vi "test Data Width and Data Loss Error.vi"(8 "error in (no error)":errorcluster, 11 "TestCase in":refnum<class "BCD.lvclass">) -> (0 "error out":errorcluster, 3 "TestCase out":refnum<class "BCD.lvclass">)   [LabVIEW 2020, in "BCD.lvclass"]
uses:
  BCD.lvclass
  e4b8c782-df88-4a73-9bfb-bbb124582f89.vi
  e994315a-18d4-4c7c-aace-f9d3bec48076.vi
  3423ebfb-ba8f-439c-a507-83e880fcea0a.vi
  5f41c702-736d-46cb-8ad7-d7a8da9834e5.vi
  e4b8c782-df88-4a73-9bfb-bbb124582f89.vi/a54b505c-1216-4ef4-8378-3ceda9d188df.vi
  e4b8c782-df88-4a73-9bfb-bbb124582f89.vi/136dcdcb-2dd3-4a4d-a796-a8f7a3f8e1ac.vi
  e994315a-18d4-4c7c-aace-f9d3bec48076.vi/0a001d06-2809-4638-8d0b-e017d2157007.vi
  BCD Decode Integer.vi
  3423ebfb-ba8f-439c-a507-83e880fcea0a.vi/a54b505c-1216-4ef4-8378-3ceda9d188df.vi
  3423ebfb-ba8f-439c-a507-83e880fcea0a.vi/136dcdcb-2dd3-4a4d-a796-a8f7a3f8e1ac.vi
  5f41c702-736d-46cb-8ad7-d7a8da9834e5.vi/a54b505c-1216-4ef4-8378-3ceda9d188df.vi
  5f41c702-736d-46cb-8ad7-d7a8da9834e5.vi/136dcdcb-2dd3-4a4d-a796-a8f7a3f8e1ac.vi
  e4b8c782-df88-4a73-9bfb-bbb124582f89.vi/a54b505c-1216-4ef4-8378-3ceda9d188df.vi/a7fcce85-1f75-4572-aeaa-ddfd463a7c5f.vi
  BCD Decode Integer.vi/9a65bfc0-0d77-4ef3-ab58-63df1e1caa90.vi
  3423ebfb-ba8f-439c-a507-83e880fcea0a.vi/a54b505c-1216-4ef4-8378-3ceda9d188df.vi/a7fcce85-1f75-4572-aeaa-ddfd463a7c5f.vi
  5f41c702-736d-46cb-8ad7-d7a8da9834e5.vi/a54b505c-1216-4ef4-8378-3ceda9d188df.vi/a7fcce85-1f75-4572-aeaa-ddfd463a7c5f.vi
  <vilib>/addons/_JKI Toolkits/VI Tester/TestCase.llb/TestCase.lvclass
  C:/Program Files (x86)/National Instruments/LabVIEW 2020/vi.lib/addons/_JKI Toolkits/VI Tester/TestCase.llb/TestCase.lvclass
panel:
  out "BCD encoded value":bool[](array[boolean])
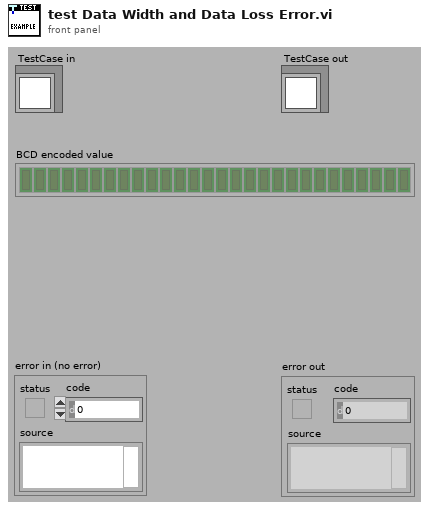
[diagram p1: front panel]
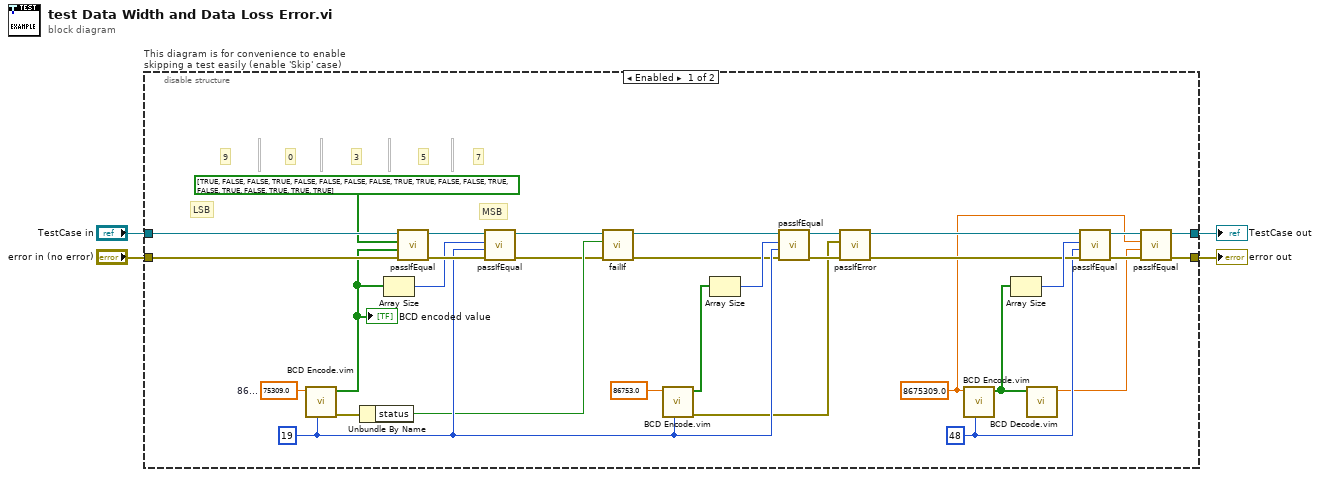
[diagram p0: block diagram]
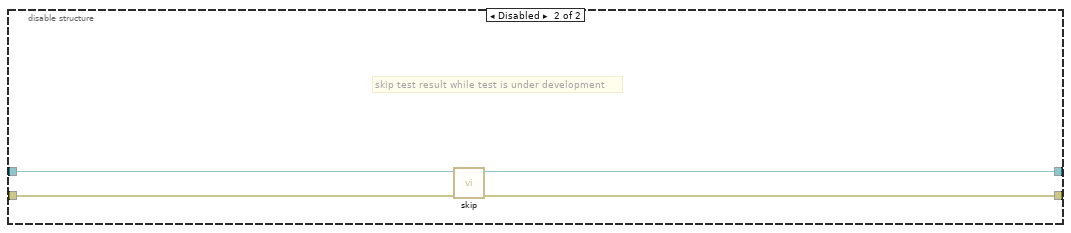
[diagram p2: hidden frame]
diagram:
  n1 = disable-structure "This diagram is for convenience to enable skipping a test easily (enable 'Skip' case)" shown="Enabled" {
    disable-tunnel: "TestCase in" -> [w35 w40]
    disable-tunnel: [w5 w38] -> w1
    disable-tunnel: [w6 w39] -> w3
    disable-tunnel: "error in (no error)" -> [w33 w37]
    frame Enabled {
      w8 = 48 ("data size (bits)")
      w9 = 8675309.0 ("86...")
      w24 = 19 ("data size (bits)")
      w27 = 75309.0  # 86...
      # "MSB"
      # "LSB"
      # "9"
      # "0"
      # "3"
      # "5"
      # "7"
      n2 = call "BCD Encode.vim"("data size (bits)"=w24, "value"=w27) -> ("error out"=w21:errorcluster, "BCD encoded value"=w29:bool[])  [unwired: 7 in, 1 out]
      "BCD encoded value" <- w29
      n3 = Unbundle By Name(w21) -> ("status"=w20:bool)
      n4 = Array Size(array=w29) -> (size(s)=w28:i32)
      n5 = call-dynamic "passIfEqual.vi"("error in (no error)"=w33, "y"=w29, "x"=bool[] [TRUE, FALSE, FALSE, TRUE, FALSE, FALSE, FALSE, FALSE, TRUE, TRUE, FALSE, FALSE, TRUE, FALSE, TRUE, FALSE, TRUE, TRUE, TRUE] ("BCD encoded value"), "TestCase in"=w35) -> ("error out"=w34:errorcluster, "TestCase out"=w36:refnum<class "BCD.lvclass">)  [unwired: 6 in]
      n6 = call-dynamic "passIfEqual.vi"("error in (no error)"=w34, "y"=w24, "x"=w28, "TestCase in"=w36) -> ("error out"=w18:errorcluster, "TestCase out"=w19:refnum<class "BCD.lvclass">)  [unwired: 6 in]
      n7 = call-dynamic "failIf.vi"("error in (no error)"=w18, "fail"=w20, "TestCase in"=w19) -> ("error out"=w16:errorcluster, "TestCase out"=w17:refnum<class "BCD.lvclass">)  [unwired: 7 in]
      n8 = call "BCD Encode.vim"("data size (bits)"=w24, "value"=86753.0 ("86...")) -> ("error out"=w22:errorcluster, "BCD encoded value"=w25:bool[])  [unwired: 7 in, 1 out]
      n9 = Array Size(array=w25) -> (size(s)=w23:i32)
      n10 = call-dynamic "passIfEqual.vi"("error in (no error)"=w16, "y"=w24, "x"=w23, "TestCase in"=w17) -> ("error out"=w31:errorcluster, "TestCase out"=w32:refnum<class "BCD.lvclass">)  [unwired: 6 in]
      n11 = call-dynamic "passIfError.vi"("error in (no error)"=w31, "error"=w22, "TestCase in"=w32) -> ("error out"=w12:errorcluster, "TestCase out"=w10:refnum<class "BCD.lvclass">)  [unwired: 7 in]
      n12 = call "BCD Encode.vim"("data size (bits)"=w8, "value"=w9) -> ("BCD encoded value"=w11:bool[])  [unwired: 7 in, 2 out]
      n13 = Array Size(array=w11) -> (size(s)=w15:i32)
      n14 = call "BCD Decode.vim"("BCD encoded value"=w11) -> ("value"=w7:dbl)  [unwired: 10 in]
      n15 = call-dynamic "passIfEqual.vi"("error in (no error)"=w12, "y"=w8, "x"=w15, "TestCase in"=w10) -> ("error out"=w14:errorcluster, "TestCase out"=w13:refnum<class "BCD.lvclass">)  [unwired: 6 in]
      n16 = call-dynamic "passIfEqual.vi"("error in (no error)"=w14, "y"=w7, "x"=w9, "TestCase in"=w13) -> ("error out"=w6:errorcluster, "TestCase out"=w5:refnum<class "BCD.lvclass">)  [unwired: 6 in]
    }
    frame Disabled {
      # "skip test result while test is under development"
      n17 = call <vilib>:"skip.vi"("error in (no error)"=w37, "TestCase in"=w40) -> ("error out"=w39:errorcluster, "TestCase out"=w38:refnum<class "BCD.lvclass">)  [unwired: 8 in]
    }
  }
  "error out" <- w3
  "TestCase out" <- w1
